vi "Write Async Queue Timeout.vi"(8 "error in":errorcluster, 10 "Queue Timeout":i32, 11 "Module Editor Node in":refnum<class "module editor node.lvclass">) -> (0 "error out":errorcluster, 3 "Module Editor Node out":refnum<class "module editor node.lvclass">)   [LabVIEW 2013, in "PL Framework Configuration Tool.lvlib" / "module editor node.lvclass"]
uses:
  module editor node.lvclass
  module editor node.lvclass/module editor node.ctl
  asynchronous execution module/configuration/asynchronous execution module configuration.lvclass/asynchronous execution module configuration.ctl
  asynchronous execution module/configuration/asynchronous execution module configuration.lvclass
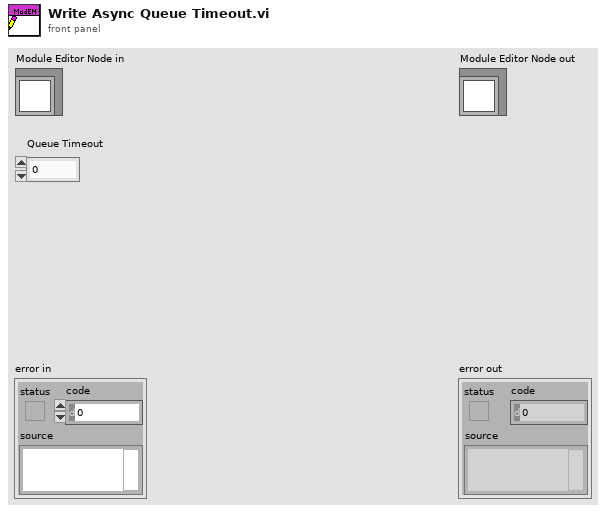
[diagram p1: front panel]
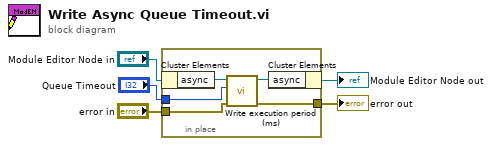
[diagram p0: block diagram]
diagram:
  n1 = in-place {
    in-place-border: "Queue Timeout" -> [w6]
    in-place-border: [w8] -> w2
    in-place-border: "error in" -> [w7]
    n2 = in-place-cluster #1("Module Editor Node in") -> ("async"=w10:refnum<class "asynchronous execution module configuration.lvclass">)
    n3 = call "Write execution period (ms).vi"("error in"=w7, "execution period (ms)"=w6, "Asynchronous Component Configuration in"=w10) -> ("error out"=w8:errorcluster, "Asynchronous Component Configuration out"=w9:refnum<class "asynchronous execution module configuration.lvclass">)  [unwired: 7 in]
    n4 = in-place-cluster #1("async"=w9) -> (→"Module Editor Node out":refnum<class "module editor node.lvclass">)
  }
  "error out" <- w2
